vi "CRYO_VavleControlProto.vi"() -> ()   [LabVIEW 2017]
uses:
  istr.lib/ADCMT 6240/Public/Configure/Configure Output Mode (DC).vi
  istr.lib/ADCMT 6240/Public/Action-Status/Output (Suspend).vi
  istr.lib/ADCMT 6240/Public/Action-Status/Output (Operate).vi
  istr.lib/ADCMT 6240/Public/Data/Read (Single Point).vi
  istr.lib/ADCMT 6240/ADCMT 6240.lvlib
panel:
  out "Initialized?":bool
  in  "Stop Button":bool
  out "Actual Voltage (V)":dbl
  out "Actual Current (mA)":dbl
  in  "Set Current (mA)":dbl(knob)=4.0 min=4.0 max=20.0 step=0.5 scale=4.0..20.0
  in  "Output ON/OFF":bool
  in  "Low Limiter Value (-0.3)":dbl=-0.3 min=-15.0 max=15.0 step=0.0001 format="%_4g"
  out "Error Out":errorcluster
  in  "Enable Auto Range":bool
  in  "Limiter Value (0.3)":dbl=0.3 min=-15.0 max=15.0 step=1.0 format="%_4g"
  in  "VISA resource name":refnum<visa-resource-name>
  in  "Initialize":bool
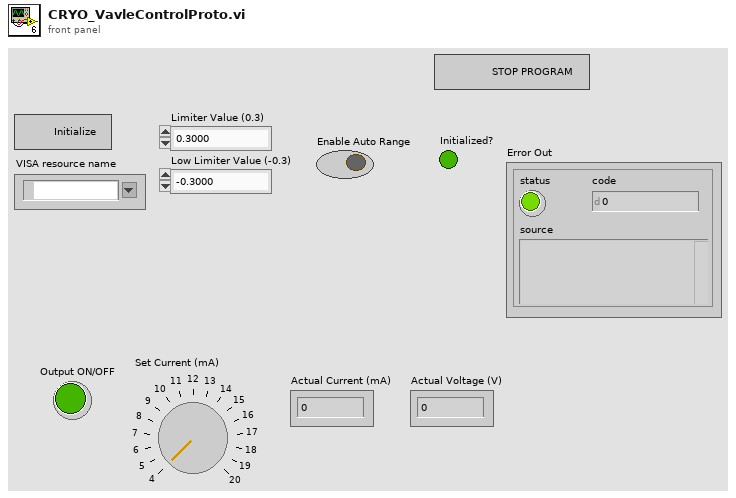
[diagram p1: front panel]
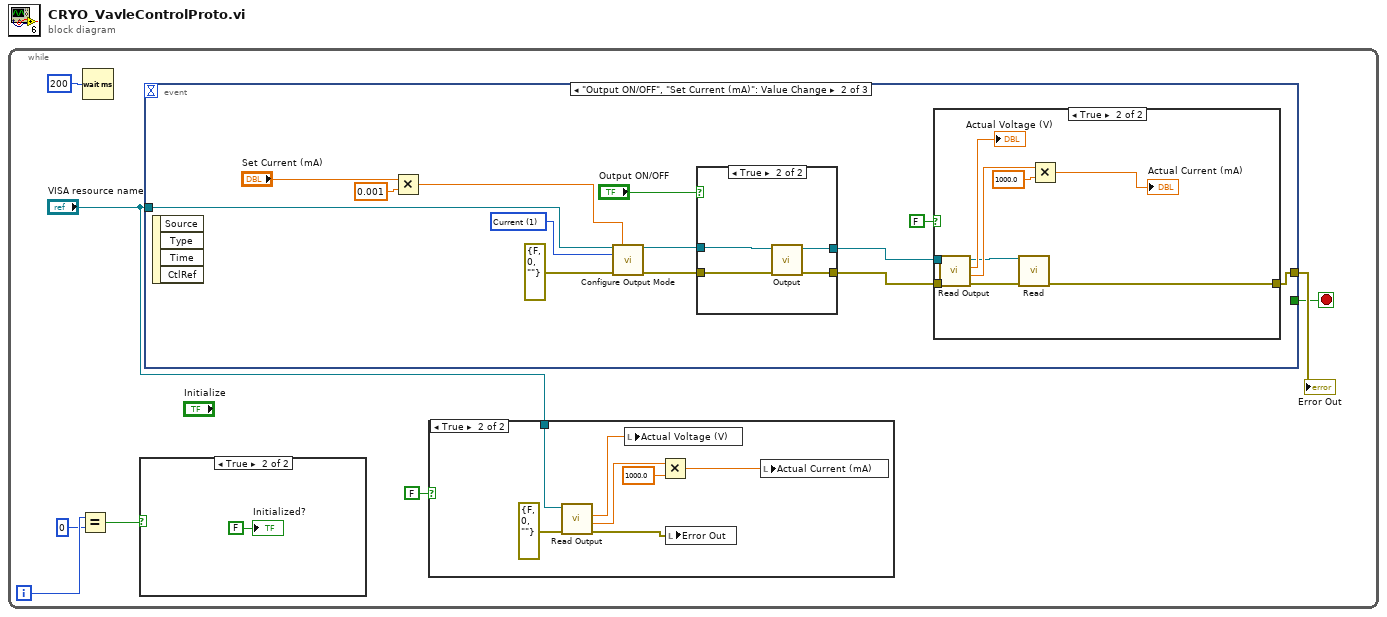
[diagram p0: block diagram]
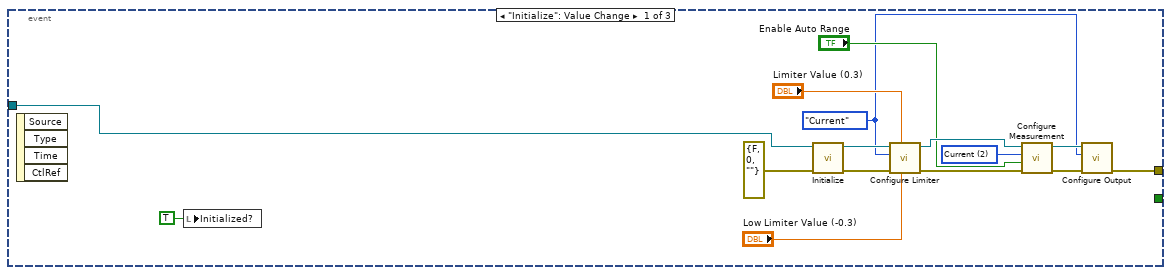
[diagram p4: hidden frame]
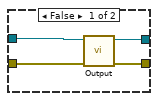
[diagram p6: hidden frame]
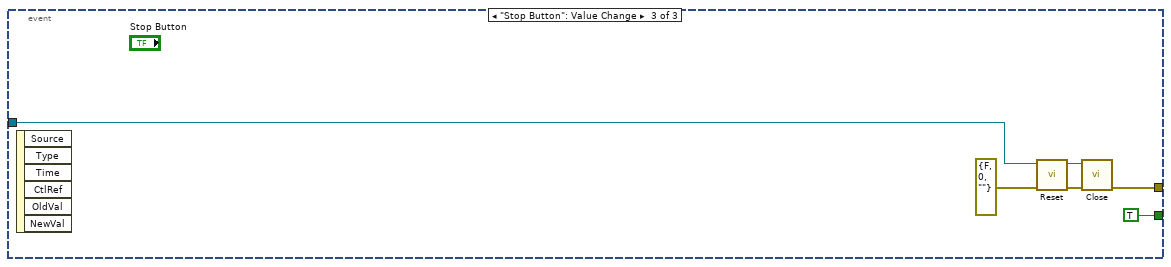
[diagram p7: hidden frame]
diagram:
  n1 = while {
    i -> [w4]
    stop <- w6 stop-if-true
    n2 = Equal?(x=w4, y=0) -> (x = y?=w2:bool)
    n3 = Wait (ms)(milliseconds to wait=u32 200) -> ()  [unwired: 1 out]
    n4 = case shown="True" w2 {
      frame False {
      }
      frame True {
        "Initialized?" <- FALSE ("Initialized?")
      }
    }
    n5 = event shown="[1] \"Output ON/OFF\", \"Set Current (mA)\": Value Change" {
      selector: _ -> [_ _ _]
      dyn-events: _ -> [_ _ _]
      timeout: _ -> [_ _ _]
      tunnel: "VISA resource name" -> [w31 w42 w66]
      tunnel: [w19 w33 w67] -> w7
      tunnel: [_ _ TRUE ("Stop Button")] -> w6
      event "Initialize": Value Change {
        w18 = enum16{"Voltage", "Current"}."Current" ("Source Function  (0: Voltage)")
        w25 = 2 items=["Off", "Volts", "Current", "Resistance"] ("Measurement Function (2: Current)")
        n6 = event-data() -> ()  [unwired: 1 in, 4 out]
        n7 = local write "Initialized?"(TRUE ("Initialized?")) -> ()
        n8 = call "Initialize.vi"("error in (no error)"=errorcluster {"status"=FALSE, "code"=0, "source"=""}, "VISA resource name"=w31) -> ("error out"=w29:errorcluster, "VISA resource name out"=w28:refnum<visa-resource-name>)  [unwired: 8 in]
        n9 = call "Configure Limiter.vi"("Low Limiter Value (-0.3)"="Low Limiter Value (-0.3)", "Limiter Value (0.3)"="Limiter Value (0.3)", "error in (no error)"=w29, "Source Function  (0: Voltage)"=w18, "VISA resource name"=w28) -> ("error out"=w24:errorcluster, "VISA resource name out"=w26:refnum<visa-resource-name>)  [unwired: 5 in]
        n10 = call "Configure Measurement.vi"("error in (no error)"=w24, "Enable Auto Range (F: Disable)"="Enable Auto Range", "Measurement Function (2: Current)"=w25, "VISA resource name"=w26) -> ("error out"=w20:errorcluster, "VISA resource name out"=w21:refnum<visa-resource-name>)  [unwired: 6 in]
        n11 = call "Configure Output.vi"("error in (no error)"=w20, "Source Function  (0: Voltage)"=w18, "VISA resource name"=w21) -> ("error out"=w19:errorcluster)  [unwired: 7 in, 1 out]
      }
      event "Output ON/OFF", "Set Current (mA)": Value Change {
        w41 = 1 items=["Voltage", "Current"] ("Source Function  (0: Voltage)")
        n12 = event-data() -> ()  [unwired: 1 in, 4 out]
        n13 = Multiply(x="Set Current (mA)", y=0.001) -> (x*y=w36:dbl)
        n14 = call-poly "Configure Output Mode.vi"("VISA resource name"=w42, "Output Value (0.0)"=w36, "Source Function  (0: Voltage)"=w41, "error in (no error)"=errorcluster {"status"=FALSE, "code"=0, "source"=""}) -> ("VISA resource name out"=w39:refnum<visa-resource-name>, "error out"=w37:errorcluster)  [unwired: 10 in]
        n15 = case shown="True" "Output ON/OFF" {
          tunnel: w39 -> [w58 w62]
          tunnel: w37 -> [w57 w61]
          tunnel: [w56 w60] -> w34
          tunnel: [w55 w59] -> w35
          frame False {
            n16 = call-poly "Output.vi"("error in (no error)"=w57, "VISA resource name"=w58) -> ("error out"=w56:errorcluster, "VISA resource name out"=w55:refnum<visa-resource-name>)  [unwired: 8 in]
          }
          frame True {
            n17 = call-poly "Output.vi"("error in (no error)"=w61, "VISA resource name"=w62) -> ("error out"=w60:errorcluster, "VISA resource name out"=w59:refnum<visa-resource-name>)  [unwired: 8 in]
          }
        }
        n18 = case shown="True" FALSE {
          tunnel: w35 -> [_ w54]
          tunnel: w34 -> [w45 w53]
          tunnel: [w45 w47] -> w33
          frame False {
          }
          frame True {
            n19 = call "Read Output.vi"("error in (no error)"=w53, "VISA resource name"=w54) -> ("error out"=w48:errorcluster, "Actual Current Level (A)"=w52:dbl, "Actual Voltage Level (V)"=→"Actual Voltage (V)":dbl, "VISA resource name out"=w46:refnum<visa-resource-name>)  [unwired: 6 in]
            n20 = call-poly "Read.vi"("VISA resource name"=w46, "error in"=w48) -> ("error out"=w47:errorcluster)  [unwired: 7 in, 6 out]
            n21 = Multiply(x=w52, y=1000.0) -> (x*y=→"Actual Current (mA)":dbl)
          }
        }
      }
      event "Stop Button": Value Change {
        n22 = event-data() -> ()  [unwired: 1 in, 6 out]
        n23 = call "Reset.vi"("error in (no error)"=errorcluster {"status"=FALSE, "code"=0, "source"=""}, "VISA resource name"=w66) -> ("error out"=w63:errorcluster, "VISA resource name out"=w64:refnum<visa-resource-name>)  [unwired: 8 in]
        n24 = call "Close.vi"("error in (no error)"=w63, "VISA resource name"=w64) -> ("error out"=w67:errorcluster)  [unwired: 9 in]
      }
    }
    "Error Out" <- w7
    n25 = case shown="True" FALSE {
      tunnel: "VISA resource name" -> [_ w11]
      frame False {
      }
      frame True {
        n26 = call "Read Output.vi"("error in (no error)"=errorcluster {"status"=FALSE, "code"=0, "source"=""}, "VISA resource name"=w11) -> ("error out"=w10:errorcluster, "Actual Current Level (A)"=w14:dbl, "Actual Voltage Level (V)"=w16:dbl)  [unwired: 6 in, 1 out]
        n27 = local write "Actual Voltage (V)"(w16) -> ()
        n28 = Multiply(x=w14, y=1000.0) -> (x*y=w15:dbl)
        n29 = local write "Error Out"(w10) -> ()
        n30 = local write "Actual Current (mA)"(w15) -> ()
      }
    }
  }
